vi "Initialize.vi"(8 "error in (no error)":errorcluster, 10 "config path":path, 11 "Quartz in":refnum<class "Quartz.lvclass">) -> (0 "error out":errorcluster, 3 "Quartz out":refnum<class "Quartz.lvclass">)   [LabVIEW 2016, in "Quartz.lvclass"]
uses:
  Quartz.lvclass
  LightBox/LightBox.lvclass
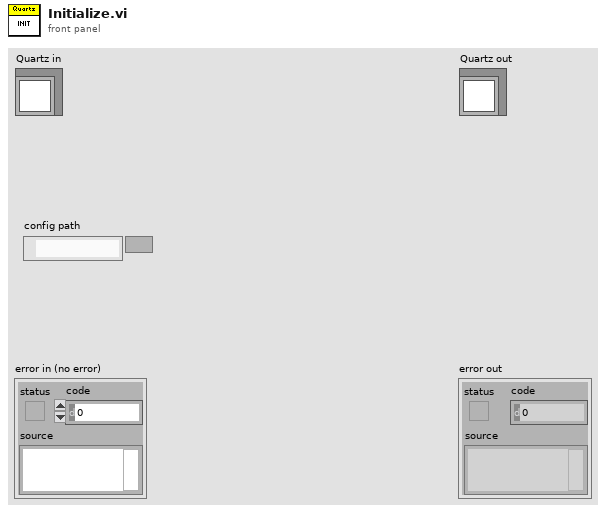
[diagram p1: front panel]
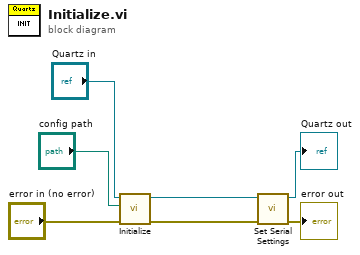
[diagram p0: block diagram]
diagram:
  n1 = call-parent "Initialize.vi"("error in (no error)"="error in (no error)", "config path"="config path", "LightBox in"="Quartz in") -> ("error out"=w2:errorcluster, "LightBox out"=w4:refnum<class "Quartz.lvclass">)  [unwired: 7 in]
  n2 = call-dynamic "Set Serial Settings.vi"("error in (no error)"=w2, "Quartz in"=w4) -> ("error out"=→"error out":errorcluster, "Quartz out"=→"Quartz out":refnum<class "Quartz.lvclass">)  [unwired: 8 in]
